vi "rethinkdb_msg_handshake_final.vi"(6 "protocol_version":i32, 8 "error in (no error)":errorcluster, 9 "client_first_message":string, 10 "password":string, 11 "server_response (json)":string="{\"success\":true,\"min_protocol_version\":0,\"max_protocol_version\":0,\"server_version\":\"2.3.0\"}\u0000\n{\"success\":true,\"authentication\":\"r=rOprNGfwEbeRWgbNEkqO%hvYDpWUa2RaTCAfuxFIlj)hNlF$k0,s=W22ZaJ0SNY7soEsUEjb6gQ==,i=4096\"}\u0000") -> (0 "error out":errorcluster, 3 "authentication_request":string)   [LabVIEW 2017]
uses:
  607e8d35-8043-420e-ade6-b7108c8a96a2.vi
  c8c95386-0f90-43b3-bd9c-7c1deb51f365.vi
  c183e845-0e18-43da-aa1f-dd9aa299a331.vi
  json/json_resolve_key.vi
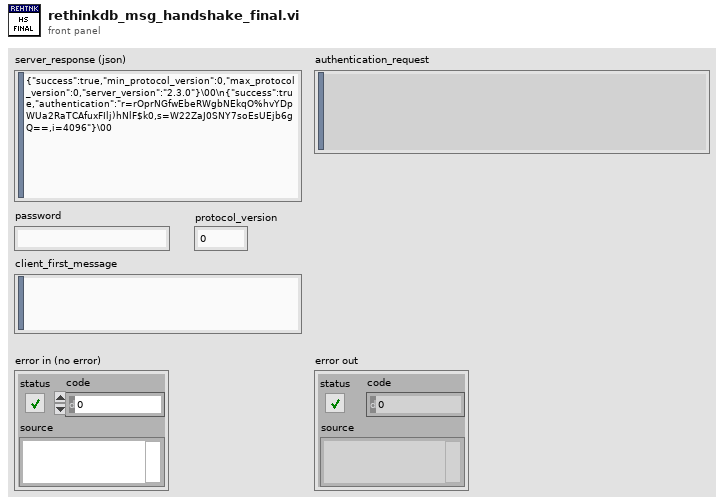
[diagram p1: front panel]
types:
  T1 = typedef "json_element.ctl" = cluster{"path":string, "type":T2, "value":variant}
  T2 = typedef "json_element_type.ctl" = enum8{"null", "bool", "int", "uint", "float", "string", "array", "object"}
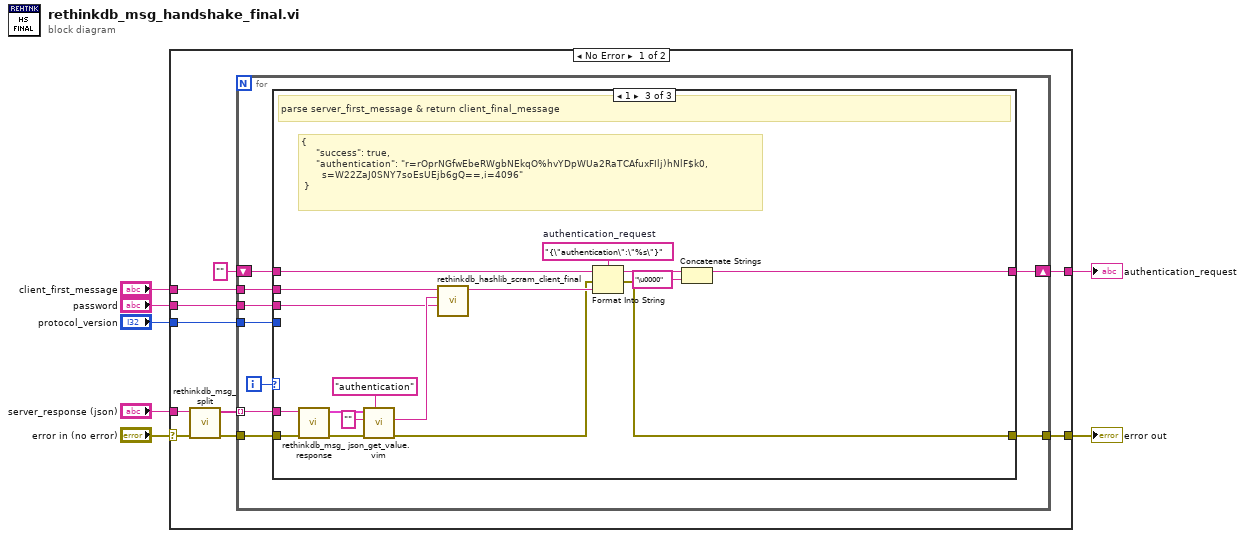
[diagram p0: block diagram]
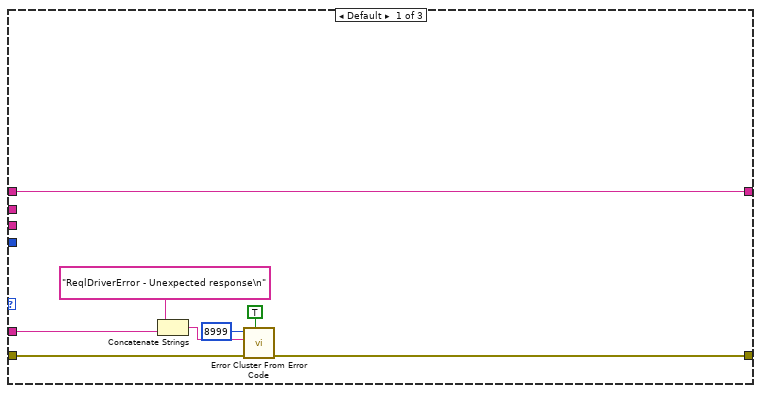
[diagram p2: hidden frame]
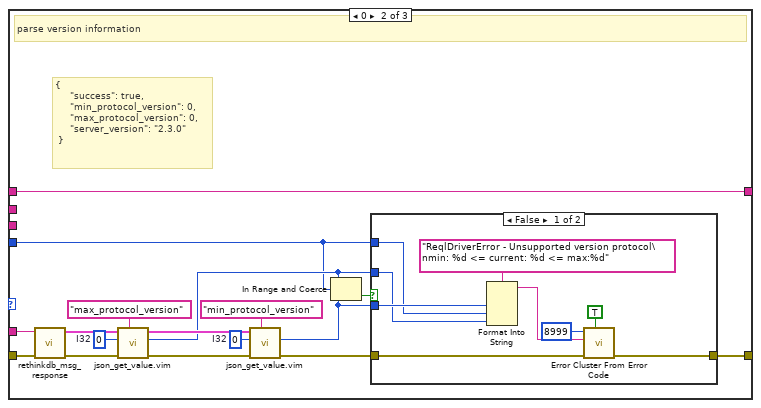
[diagram p3: hidden frame]
diagram:
  n1 = case shown="No Error" "error in (no error)" {
    selector: "error in (no error)" -> [w17 w79]
    tunnel: [w15 w79] -> w6
    tunnel: [w14 _] -> w5
    tunnel: "server_response (json)" -> [w16 _]
    tunnel: "client_first_message" -> [w12 _]
    tunnel: "password" -> [w11 _]
    tunnel: "protocol_version" -> [w8 _]
    frame No Error {
      n2 = call "rethinkdb_msg_split.vi"("error in (no error)"=w17, "data in"=w16) -> ("error out"=w10:errorcluster, "messages"=w13:string[])  [unwired: 7 in, 1 out]
      n3 = for {
        tunnel: [w26] -> w15
        tunnel: w13 -> [w21] mode=indexing
        tunnel: w11 -> [w23]
        tunnel: w10 -> [w22]
        tunnel: w12 -> [w24]
        shift-right: [w25] -> w14
        shift-left: "" -> [w19]
        tunnel: w8 -> [w18]
        i -> [w20]
        n4 = case shown="1" w20 {
          tunnel: [w28 w40 w78] -> w26
          tunnel: [w27 w42 w77] -> w25
          tunnel: w24 -> [_ _ w68]
          tunnel: w23 -> [_ _ w67]
          tunnel: w22 -> [w30 w51 w66]
          tunnel: w21 -> [w29 w43 w65]
          tunnel: w19 -> [w27 w42 w62]
          tunnel: w18 -> [_ w35 _]
          frame Default {
            n5 = Concatenate Strings("ReqlDriverError - Unexpected response\n" ("error message (\"\")"), w29) -> (w31:string)
            n6 = call <vilib>:"Error Cluster From Error Code.vi"("show call chain? (False)"=TRUE, "error in (no error)"=w30, "error message (\"\")"=w31, "error code (0)"=8999) -> ("error out"=w28:errorcluster)  [unwired: 5 in]
          }
          frame 0 {
            w41 = 0  # I32
            w44 = 0  # I32
            # "{\n     \"success\": true,\n     \"min_protocol_version\": 0,\n     \"max_protocol_version\": 0,\n     \"server_version\": \"2.3.0\"\n }"
            # "parse version information"
            n7 = call "rethinkdb_msg_response.vi"("error in (no error)"=w51, "response"=w43) -> ("error out"=w49:errorcluster, "elements"=w48:T1[])  [unwired: 8 in]
            n8 = call "json_get_value.vim"("key"="max_protocol_version", "error in (no error)"=w49, "default"=w44, "elements in"=w48) -> ("error out"=w45:errorcluster, "value"=w36:i32, "elements out"=w46:T1[])  [unwired: 4 in, 1 out]
            n9 = call "json_get_value.vim"("key"="min_protocol_version", "error in (no error)"=w45, "default"=w41, "elements in"=w46) -> ("error out"=w39:errorcluster, "value"=w37:i32)  [unwired: 4 in, 2 out]
            n10 = In Range and Coerce(upper limit=w36, x=w35, lower limit=w37) -> (In Range?=w38:bool)  [unwired: 1 out]
            n11 = case shown="False" w38 {
              tunnel: [w57 w61] -> w40
              tunnel: w39 -> [w58 w61]
              tunnel: w37 -> [w56 _]
              tunnel: w35 -> [w53 _]
              tunnel: w36 -> [w52 _]
              frame False {
                n12 = Format Into String(format string="ReqlDriverError - Unsupported version protocol\nmin: %d <= current: %d <= max:%d" ("error message (\"\")"), w56, w53, w52) -> (resulting string=w54:string)  [unwired: 2 in, 1 out]
                n13 = call <vilib>:"Error Cluster From Error Code.vi"("show call chain? (False)"=TRUE, "error in (no error)"=w58, "error message (\"\")"=w54, "error code (0)"=8999) -> ("error out"=w57:errorcluster)  [unwired: 5 in]
              }
              frame True {
                # "supported protocol version"
              }
            }
          }
          frame 1 {
            w76 = "{\"authentication\":\"%s\"}"  # authentication_request
            # "{\n     \"success\": true,\n     \"authentication\": \"r=rOprNGfwEbeRWgbNEkqO%hvYDpWUa2RaTCAfuxFIlj)hNlF$k0,\n       s=W22ZaJ0SNY7soEsUEjb6gQ==,i=4096\"\n }"
            # "parse server_first_message & return client_final_message"
            n14 = call "rethinkdb_msg_response.vi"("error in (no error)"=w66, "response"=w65) -> ("error out"=w63:errorcluster, "elements"=w64:T1[])  [unwired: 8 in]
            n15 = call "json_get_value.vim"("key"="authentication", "error in (no error)"=w63, "default"="", "elements in"=w64) -> ("error out"=w70:errorcluster, "value"=w69:string)  [unwired: 4 in, 2 out]
            n16 = call "rethinkdb_hashlib_scram_client_final.vi"("password"=w67, "server_first_message"=w69, "client_first_message"=w68) -> ("client_final_message"=w71:string)  [unwired: 8 in]
            n17 = Format Into String(format string=w76, initial string=w62, error in=w70, w71) -> (resulting string=w75:string, error out=w78:errorcluster)
            n18 = Concatenate Strings(w75, "\u0000" ("string")) -> (w77:string)
          }
        }
      }
    }
    frame Error {
    }
  }
  "error out" <- w6
  "authentication_request" <- w5
